vi "Temp Matrix Update.vi"(5 "Property Name":T9, 6 "State":T10=enum."Update Graph", 7 "Data Name":T8, 8 "error in (no error)":errorcluster, 11 "Property In":variant) -> (0 "error out":errorcluster, 3 "Item Strings":string[](array[string]))   [LabVIEW 2020, in "XY Plot Matrix.lvclass"]
uses:
  <vilib>/Math Plots/2D Math Plots/XY Plot Matrix/XY Plot Matrix/XY Plot Matrix.lvclass
  <vilib>/Math Plots/2D Math Plots/2D Plot/2D Plot/Typedef/Graph General Property.ctl
  <vilib>/Math Plots/2D Math Plots/2D Plot/2D Plot/Typedef/Scale Array.ctl
  <vilib>/Math Plots/2D Math Plots/2D Plot/2D Plot/Typedef/Scale Cluster.ctl
  <vilib>/Utility/miscctls.llb/LVOffsetAndMultiplierTypeDef.ctl
  <vilib>/Math Plots/2D Math Plots/2D Plot/2D Plot/Typedef/Temp Graph State.ctl
  <vilib>/Math Plots/2D Math Plots/2D Plot/2D Plot/Typedef/Temp Graph Property Action.ctl
  <vilib>/Math Plots/2D Math Plots/2D Plot/2D Plot/Typedef/Temp Graph Data Action.ctl
  <vilib>/Math Plots/2D Math Plots/XY Plot Matrix/XY Plot Matrix/Typedef/Plotmatrix Property Array.ctl
  <vilib>/Math Plots/2D Math Plots/XY Plot Matrix/XY Plot Matrix/Typedef/Plotmatrix Property.ctl
  <vilib>/Math Plots/2D Math Plots/2D Plot/2D Plot/Typedef/Plot Property Array.ctl
  <vilib>/Math Plots/2D Math Plots/2D Plot/2D Plot/Typedef/Plot Property.ctl
  <vilib>/Math Plots/2D Math Plots/XY Plot Matrix/XY Plot Matrix/Typedef/Mulitmatrix Representation.ctl
  <vilib>/Math Plots/2D Math Plots/XY Plot Matrix/XY Plot Matrix/Typedef/Matrix Representation.ctl
  <vilib>/Math Plots/2D Math Plots/2D Plot/2D Plot/Typedef/Range Cluster.ctl
  e:/builds/penguin/labview/branches/2020/dev/dist/vi.lib/Math Plots/2D Math Plots/2D Plot/2D Plot/2D Plot.lvclass
  <vilib>/Math Plots/2D Math Plots/2D Plot/Action String/XYPlotMatrix Ctrl Act Queue.ctl
  <vilib>/Math Plots/2D Math Plots/2D Plot/Action String/XYPlotMatrix Ctrl Act Cluster.ctl
  <vilib>/Math Plots/2D Math Plots/2D Plot/Action String/2DMathPlot State Class.ctl
  <vilib>/Math Plots/2D Math Plots/XY Plot Matrix/XY Plot Matrix/XY Plot Matrix.lvclass/XY Plot Matrix.ctl
  <vilib>/Math Plots/2D Math Plots/2D Plot/2D Plot/2D Plot.lvclass
panel:
  in  "Multimatrix Representation":T1
  in  "Plotmatrix Property Array":T4=[[{"Plot Property Array"=[{"Bar Plot Style"=0, "DigitalLineStyle"=1, "TransitionLocation"=2, "Transition Type"=0, "Fill To"=-1, "Fill/Pt. Color"=0, "Label Style"=3, "Line Style"=0, "Line Width"=0, "Plot Color"=0, "Plot Interpolation"=0, "Plot Name"="Plot 0", "Point Style"=1, "Visible?"=TRUE, "XScaleIdx"=0, "YScaleIdx"=0}]}]]
  in  "Scale Array":T11
  in  "Format Property":string[](array[string])
  in  "Graph General":T14
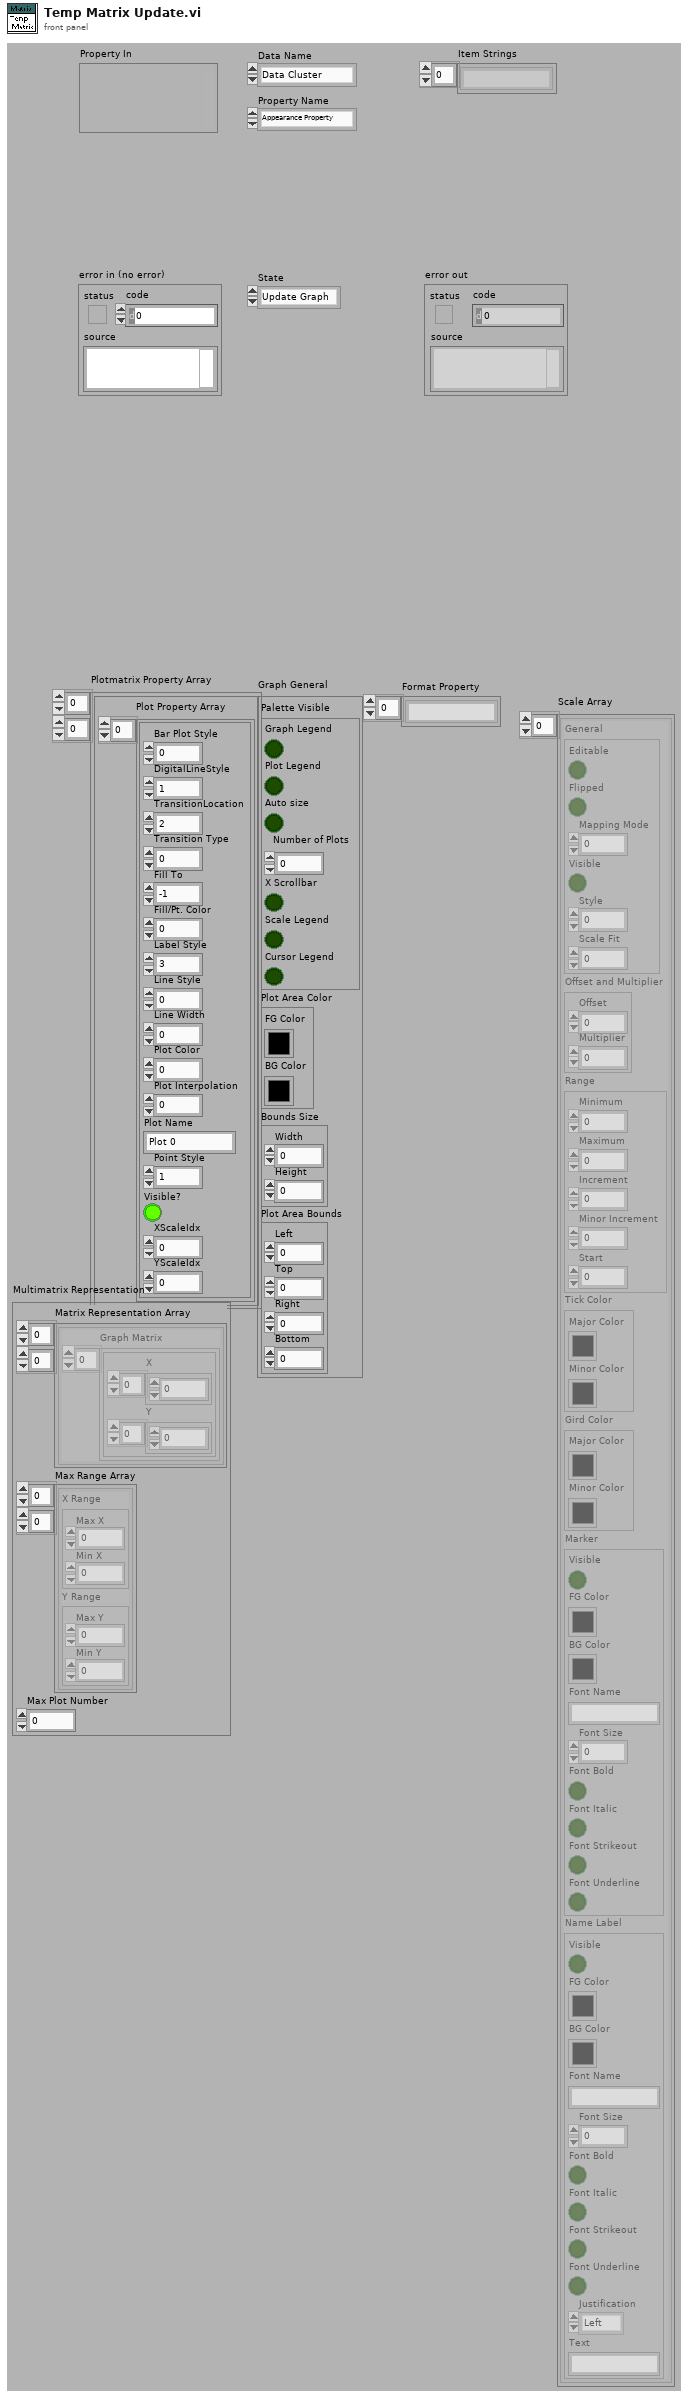
[diagram p1: front panel]
types:
  T1 = typedef "XY Plot Matrix.lvclass/Mulitmatrix Representation.ctl" = cluster{"Matrix Representation Array":T2[][], "Max Range Array":T3[][], "Max Plot Number":i32}
  T2 = typedef "XY Plot Matrix.lvclass/Matrix Representation.ctl" = cluster{"Graph Matrix":cluster{"X":dbl[], "Y":dbl[]}[]}
  T3 = typedef "2D Plot.lvclass/Range Cluster.ctl" = cluster{"X Range":cluster{"Max X":dbl, "Min X":dbl}, "Y Range":cluster{"Max Y":dbl, "Min Y":dbl}}
  T4 = typedef "XY Plot Matrix.lvclass/Plotmatrix Property Array.ctl" = T5[][]
  T5 = typedef "XY Plot Matrix.lvclass/Plotmatrix Property.ctl" = cluster{"Plot Property Array":T6}
  T6 = typedef "2D Plot.lvclass/Plot Property Array.ctl" = T7[]
  T7 = typedef "2D Plot.lvclass/Plot Property.ctl" = cluster{"Bar Plot Style":u8, "DigitalLineStyle":u8, "TransitionLocation":u8, "Transition Type":u8, "Fill To":i16, "Fill/Pt. Color":u32, "Label Style":u8, "Line Style":u8, "Line Width":u8, "Plot Color":u32, "Plot Interpolation":u8, "Plot Name":string, "Point Style":u8, "Visible?":bool, "XScaleIdx":u32, "YScaleIdx":u32}
  T8 = typedef "2D Plot.lvclass/Temp Graph Data Action.ctl" = enum16{"Data Cluster", "Property Class", "Control Queue"}
  T9 = typedef "2D Plot.lvclass/Temp Graph Property Action.ctl" = enum16{"Appearance Property", "Format Property", "Plots Property", "Scales Property"}
  T10 = typedef "2D Plot.lvclass/Temp Graph State.ctl" = enum16{"Create", "Update Graph", "Update Property Only", "Get Plot Name", "Get Axis Name", "Destory"}
  T11 = typedef "2D Plot.lvclass/Scale Array.ctl" = T12[]
  T12 = typedef "2D Plot.lvclass/Scale Cluster.ctl" = cluster{"General":cluster{"Editable":bool, "Flipped":bool, "Mapping Mode":u8, "Visible":bool, "Style":u8, "Scale Fit":u8}, "Offset and Multiplier":T13, "Range":cluster{"Minimum":dbl, "Maximum":dbl, "Increment":dbl, "Minor Increment":dbl, "Start":dbl}, "Tick Color":cluster{"Major Color":u32, "Minor Color":u32}, "Gird Color":cluster{"Major Color":u32, "Minor Color":u32}, "Marker":cluster{"Visible":bool, "FG Color":u32, "BG Color":u32, "Font Name":string, "Font Size":u32, "Font Bold":bool, "Font Italic":bool, "Font Strikeout":bool, "Font Underline":bool}, "Name Label":cluster{"Visible":bool, "FG Color":u32, "BG Color":u32, "Font Name":string, "Font Size":u32, "Font Bold":bool, "Font Italic":bool, "Font Strikeout":bool, "Font Underline":bool, "Justification":enum16{"Left", "Center", "Right"}, "Text":string}}
  T13 = typedef "LVOffsetAndMultiplierTypeDef.ctl" = cluster{"Offset":dbl, "Multiplier":dbl}
  T14 = typedef "2D Plot.lvclass/Graph General Property.ctl" = cluster{"Palette Visible":cluster{"Graph Legend":bool, "Plot Legend":bool, "Auto size":bool, "Number of Plots":u32, "X Scrollbar":bool, "Scale Legend":bool, "Cursor Legend":bool}, "Plot Area Color":cluster{"FG Color":u32, "BG Color":u32}, "Bounds Size":cluster{"Width":u32, "Height":u32}, "Plot Area Bounds":cluster{"Left":i16, "Top":i16, "Right":i16, "Bottom":i16}}
  T15 = typedef "XYPlotMatrix Ctrl Act Queue.ctl" = refnum<queue>
  T16 = typedef "2DMathPlot State Class.ctl" = enum16{"Update All (Undo)", "Update General", "Update Appearance", "Update Format", "Update Scale", "Update Marker", "Update Cursor", "None"}
  T17 = typedef "2D Plot.lvclass/Property Cluster.ctl" = cluster{"Graph General":T14, "Format Property":string[], "Scale Array":T11, "Cursor Property":T18, "Annotation List":T20, "Active Cursor":i32, "Active Plot":i32}
  T18 = typedef "2D Plot.lvclass/Cursor Property.ctl" = cluster{"Cursor List":T19, "Cursor List Addtional":cluster{"Cursor Selection Color":u32, "Line Style":u8, "Line Width":u8, "Visible":bool}[]}
  T19 = typedef "LVCursorListTypeDef.ctl" = cluster{"Name":string, "Color":u32, "Style":u8, "Point Style":u8, "Name Visible":bool, "Allow Drag":bool, "Cursor Mode":u32, "Plot":i32, "Index":i32, "Position":cluster{"X":dbl, "Y":dbl}, "X Scale":u32, "Y Scale":u32, "Watch Plots":i32[], "Watch All Plots":bool, "Plot Area":i32, "Label Offset":cluster{"X":dbl, "Y":dbl}}[]
  T20 = typedef "LVAnnotationListTypeDef.ctl" = cluster{"Name":string, "Color":u32, "Style":u8, "Point Style":u8, "Name Visible":bool, "Allow Drag":bool, "Annotation Mode":u32, "Plot":i32, "Index":i32, "Position":cluster{"X":dbl, "Y":dbl}, "X Scale":u32, "Y Scale":u32, "Show Arrow":bool, "Lock Name":bool, "Plot Area":i32, "Label Offset":cluster{"X":dbl, "Y":dbl}}[]
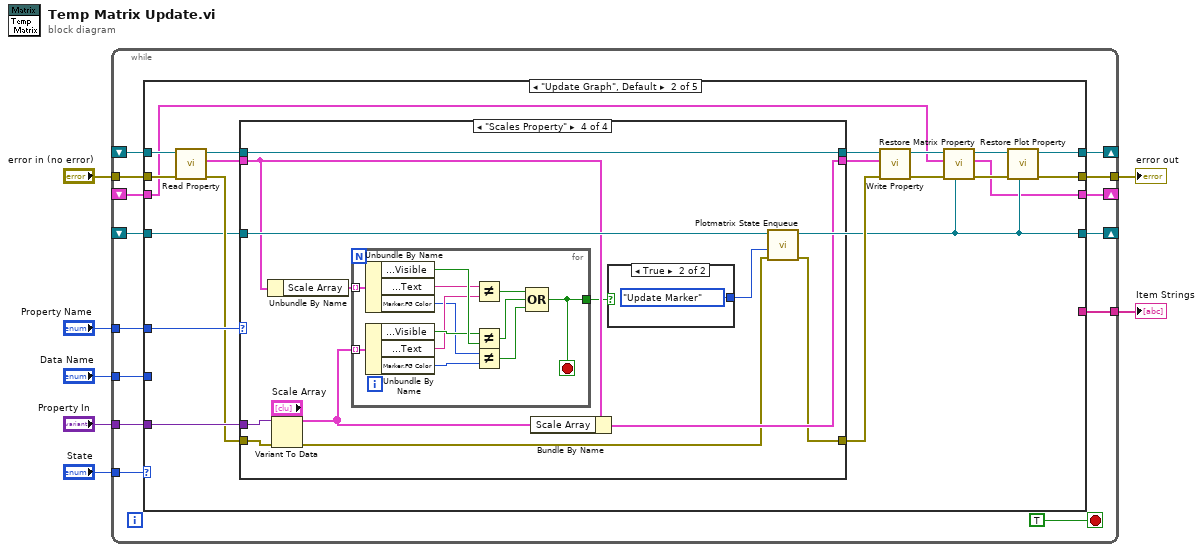
[diagram p0: block diagram]
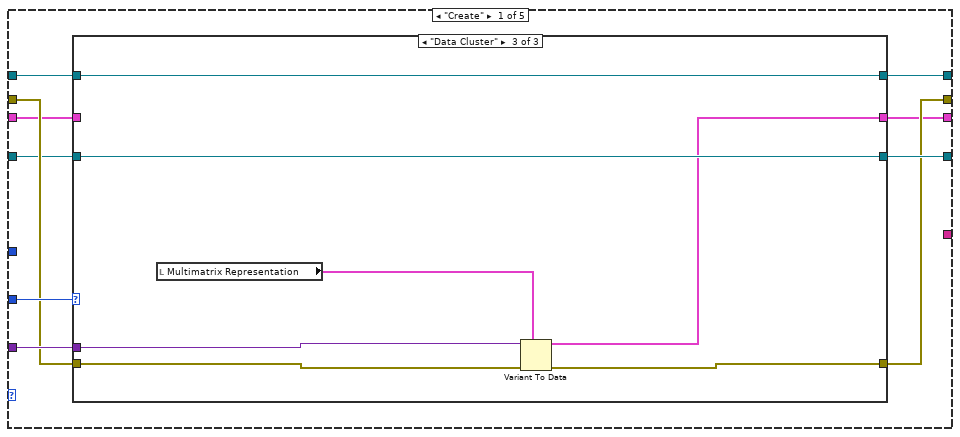
[diagram p2: hidden frame]
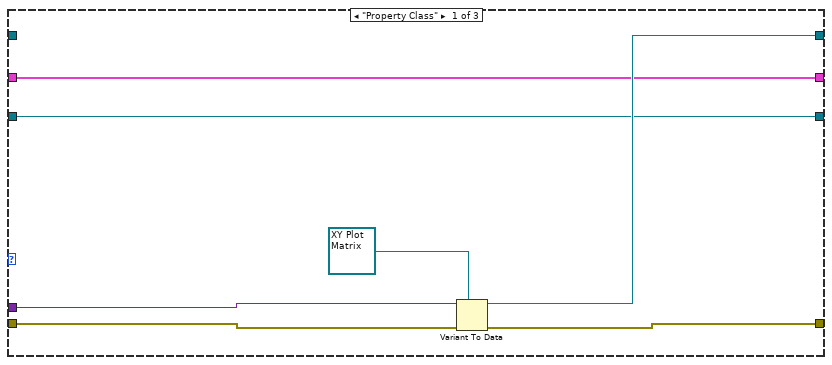
[diagram p3: hidden frame]
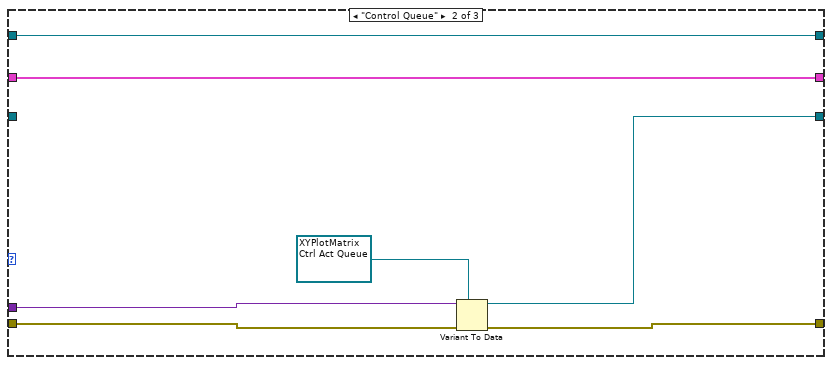
[diagram p4: hidden frame]
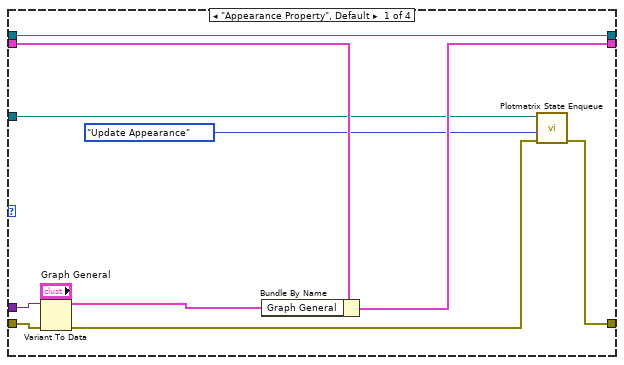
[diagram p5: hidden frame]
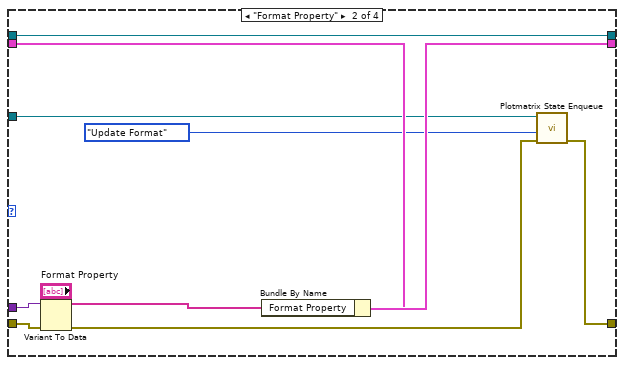
[diagram p6: hidden frame]
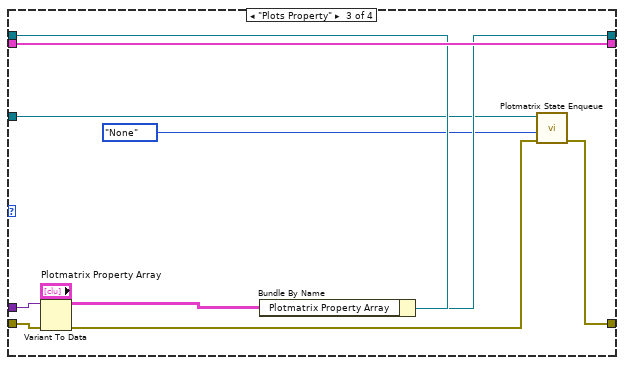
[diagram p7: hidden frame]
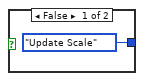
[diagram p8: hidden frame]
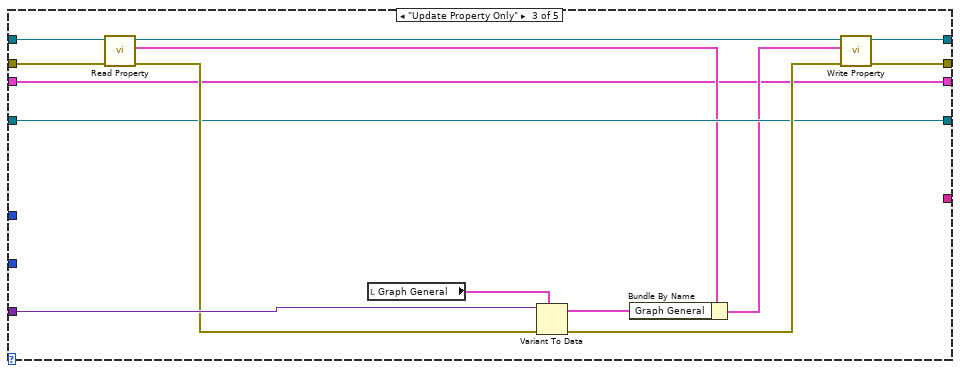
[diagram p9: hidden frame]
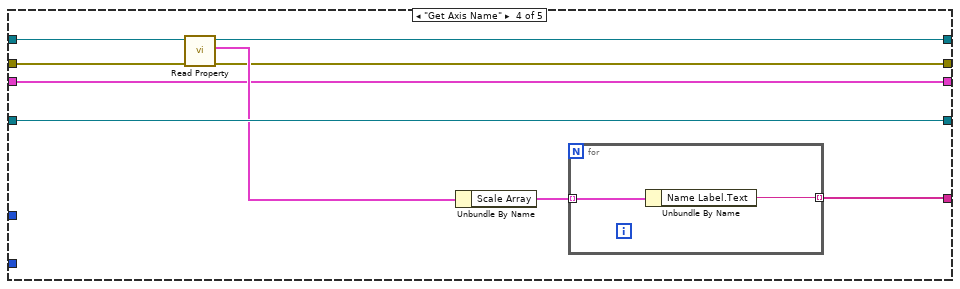
[diagram p10: hidden frame]
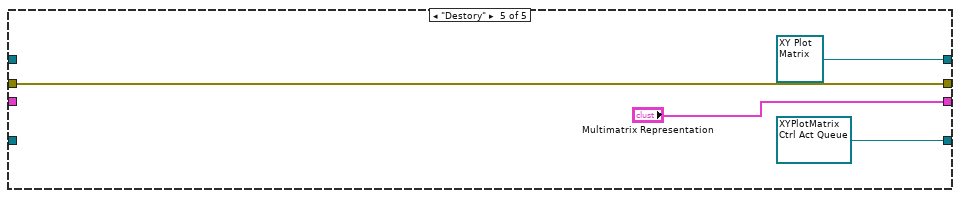
[diagram p11: hidden frame]
diagram:
  n1 = while {
    tunnel: "State" -> [w21]
    tunnel: "Property In" -> [w20]
    tunnel: "Property Name" -> [w19]
    tunnel: "Data Name" -> [w18]
    tunnel: "error in (no error)" -> [w17]
    tunnel: [w16] -> w2
    shift-right: [w14] -> _
    shift-left: _ -> [w13]
    shift-right: [w15] -> _
    shift-left: _ -> [w12]
    tunnel: [w10] -> w1
    shift-right: [w9] -> _
    shift-left: _ -> [w8]
    stop <- TRUE stop-if-true
    n2 = case shown="\"Update Graph\", Default" w21 {
      tunnel: w20 -> [w30 w71 w139 _ _]
      tunnel: w19 -> [_ w70 _ _ _]
      tunnel: w18 -> [w31 _ _ _ _]
      tunnel: w17 -> [w29 w57 w142 w148 w159]
      tunnel: [w24 w66 w141 w147 w159] -> w16
      tunnel: [w26 w67 w143 w149 refnum<class "XY Plot Matrix.lvclass"> refnum ("2D Plotmatrix.lvclass out")] -> w15
      tunnel: [w25 w55 w136 w154 T15 refnum ("Control Ref Queue")] -> w14
      tunnel: w13 -> [w27 w55 w136 w154 _]
      tunnel: w12 -> [w28 w65 w145 w150 _]
      tunnel: [_ _ _ w152 _] -> w10
      tunnel: [w23 w53 w132 w146 "Multimatrix Representation"] -> w9
      tunnel: w8 -> [w22 w54 w132 w146 _]
      frame "Create" {
        n3 = case shown="\"Data Cluster\"" w31 {
          tunnel: w30 -> [w38 w45 w49]
          tunnel: w29 -> [w37 w44 w48]
          tunnel: w28 -> [_ w41 w52]
          tunnel: w27 -> [w35 _ w51]
          tunnel: [w36 w41 w52] -> w26
          tunnel: [w35 w42 w51] -> w25
          tunnel: [w33 w40 w47] -> w24
          tunnel: [w32 w39 w46] -> w23
          tunnel: w22 -> [w32 w39 _]
          frame "Property Class" {
            n4 = Variant To Data(error in=w37, type=refnum<class "XY Plot Matrix.lvclass"> refnum ("2D Plotmatrix.lvclass"), Variant=w38) -> (data=w36:refnum<class "XY Plot Matrix.lvclass">, error out=w33:errorcluster)
          }
          frame "Control Queue" {
            n5 = Variant To Data(error in=w44, type=T15 refnum ("Control Ref Queue"), Variant=w45) -> (data=w42:T15, error out=w40:errorcluster)
          }
          frame "Data Cluster" {
            n6 = local read "Multimatrix Representation"() -> (w50:T1)
            n7 = Variant To Data(error in=w48, type=w50, Variant=w49) -> (data=w46:T1, error out=w47:errorcluster)
          }
        }
      }
      frame "Update Graph", Default {
        n8 = call <vilib>:"Read Property.vi"("error in (no error)"=w57, "2D Plot.lvclass in"=w65) -> ("error out"=w56:errorcluster, "XY Graph Property Cluster"=w62:T17, "2D Plot.lvclass out"=w64:refnum<class "XY Plot Matrix.lvclass">)  [unwired: 7 out]
        n9 = case shown="\"Scales Property\"" w70 {
          tunnel: w71 -> [w81 w93 w104 w117]
          tunnel: w56 -> [w82 w92 w103 w116]
          tunnel: [w72 w83 w95 w110] -> w59
          tunnel: w64 -> [w76 w87 w101 w113]
          tunnel: [w80 w89 w102 w115] -> w58
          tunnel: w62 -> [w77 w88 w102 w107]
          tunnel: [w76 w87 w100 w113] -> w61
          tunnel: w55 -> [w74 w85 w97 w109]
          frame "Appearance Property", Default {
            n10 = Variant To Data(error in=w82, type="Graph General", Variant=w81) -> (data=w78:T14, error out=w73:errorcluster)
            n11 = Bundle By Name(cluster=w77, "Graph General"=w78) -> (w80:T17)
            n12 = call <vilib>:"Plotmatrix State Enqueue.vi"("error in (no error)"=w73, "Display State Change Class"=2DMathPlot_State_Class."Update Appearance", "Control Ref Queue"=w74) -> ("error out"=w72:errorcluster)  [unwired: 8 out]
          }
          frame "Format Property" {
            n13 = Variant To Data(error in=w92, type="Format Property", Variant=w93) -> (data=w91:string[], error out=w84:errorcluster)
            n14 = Bundle By Name(cluster=w88, "Format Property"=w91) -> (w89:T17)
            n15 = call <vilib>:"Plotmatrix State Enqueue.vi"("error in (no error)"=w84, "Display State Change Class"=2DMathPlot_State_Class."Update Format", "Control Ref Queue"=w85) -> ("error out"=w83:errorcluster)  [unwired: 8 out]
          }
          frame "Plots Property" {
            n16 = Variant To Data(error in=w103, type="Plotmatrix Property Array", Variant=w104) -> (data=w99:T4, error out=w96:errorcluster)
            n17 = Bundle By Name(cluster=w101, "Plotmatrix Property Array"=w99) -> (w100:refnum<class "XY Plot Matrix.lvclass">)
            n18 = call <vilib>:"Plotmatrix State Enqueue.vi"("error in (no error)"=w96, "Display State Change Class"=2DMathPlot_State_Class."None", "Control Ref Queue"=w97) -> ("error out"=w95:errorcluster)  [unwired: 8 out]
          }
          frame "Scales Property" {
            n19 = Unbundle By Name(w107) -> ("Scale Array"=w106:T11)
            n20 = Variant To Data(error in=w116, type="Scale Array", Variant=w117) -> (data=w108:T11, error out=w111:errorcluster)
            n21 = for {
              tunnel: w108 -> [w130] mode=indexing
              tunnel: w106 -> [w131] mode=indexing
              tunnel: [w123] -> w105
              stop <- w123 stop-if-true
              n22 = Unbundle By Name(w131) -> ("Name Label.Visible"=w129:bool, "Name Label.Text"=w127:string, "Marker.FG Color"=w122:u32)
              n23 = Unbundle By Name(w130) -> ("Name Label.Visible"=w128:bool, "Name Label.Text"=w126:string, "Marker.FG Color"=w121:u32)
              n24 = Not Equal?(x=w127, y=w126) -> (x != y?=w125:bool)
              n25 = Not Equal?(x=w128, y=w129) -> (x != y?=w124:bool)
              n26 = Not Equal?(x=w122, y=w121) -> (x != y?=w120:bool)
              n27 = Compound Arithmetic op=OR(w125, w124, w120) -> (w123:bool)
            }
            n28 = Bundle By Name(cluster=w107, "Scale Array"=w108) -> (w115:T17)
            n29 = case shown="True" w105 {
              tunnel: [2DMathPlot_State_Class."Update Scale" ("Display State Change Class") 2DMathPlot_State_Class."Update Marker" ("Display State Change Class")] -> w112
              frame False {
              }
              frame True {
              }
            }
            n30 = call <vilib>:"Plotmatrix State Enqueue.vi"("error in (no error)"=w111, "Display State Change Class"=w112, "Control Ref Queue"=w109) -> ("error out"=w110:errorcluster)  [unwired: 8 out]
          }
        }
        n31 = call <vilib>:"Write Property.vi"("error in (no error)"=w59, "XY Graph Property Cluster"=w58, "2D Plot.lvclass in"=w61) -> ("error out"=w60:errorcluster, "2D Plot.lvclass out"=w63:refnum<class "XY Plot Matrix.lvclass">)  [unwired: 7 out]
        n32 = call <vilib>:"Restore Matrix Property.vi"("Control Ref Queue"=w55, "error in (no error)"=w60, "Matrix Representation Array In"=w54, "2D Plotmatrix.lvclass in"=w63) -> ("error out"=w69:errorcluster, "Matrix Representation Array Out"=w53:T1, "2D Plotmatrix.lvclass out"=w68:refnum<class "XY Plot Matrix.lvclass">)  [unwired: 5 out]
        n33 = call <vilib>:"Restore Plot Property.vi"("Control Ref Queue"=w55, "error in (no error)"=w69, "2D Plotmatrix.lvclass in"=w68) -> ("error out"=w66:errorcluster, "2D Plotmatrix.lvclass out"=w67:refnum<class "XY Plot Matrix.lvclass">)  [unwired: 7 out]
      }
      frame "Update Property Only" {
        n34 = call <vilib>:"Read Property.vi"("error in (no error)"=w142, "2D Plot.lvclass in"=w145) -> ("error out"=w138:errorcluster, "XY Graph Property Cluster"=w134:T17, "2D Plot.lvclass out"=w144:refnum<class "XY Plot Matrix.lvclass">)  [unwired: 7 out]
        n35 = local read "Graph General"() -> (w135:T14)
        n36 = Variant To Data(error in=w138, type=w135, Variant=w139) -> (data=w140:T14, error out=w137:errorcluster)
        n37 = Bundle By Name(cluster=w134, "Graph General"=w140) -> (w133:T17)
        n38 = call <vilib>:"Write Property.vi"("error in (no error)"=w137, "XY Graph Property Cluster"=w133, "2D Plot.lvclass in"=w144) -> ("error out"=w141:errorcluster, "2D Plot.lvclass out"=w143:refnum<class "XY Plot Matrix.lvclass">)  [unwired: 7 out]
      }
      frame "Get Axis Name" {
        n39 = call <vilib>:"Read Property.vi"("error in (no error)"=w148, "2D Plot.lvclass in"=w150) -> ("error out"=w147:errorcluster, "XY Graph Property Cluster"=w151:T17, "2D Plot.lvclass out"=w149:refnum<class "XY Plot Matrix.lvclass">)  [unwired: 7 out]
        n40 = Unbundle By Name(w151) -> ("Scale Array"=w153:T11)
        n41 = for {
          tunnel: w153 -> [w156] mode=indexing
          tunnel: [w155] -> w152 mode=indexing
          n42 = Unbundle By Name(w156) -> ("Name Label.Text"=w155:string)
        }
      }
      frame "Destory" {
      }
    }
  }
  "error out" <- w2
  "Item Strings" <- w1
